vi "Write Command.vi"(8 "Error In":errorcluster, 10 "Command":string, 11 "SerialComm in":refnum<class "SerialComm.lvclass">) -> (0 "Error Out":errorcluster, 3 "SerialComm out":refnum<class "SerialComm.lvclass">)   [LabVIEW 2016, in "SerialComm.lvclass"]
uses:
  SerialComm.lvclass
  SerialComm.lvclass/SerialComm.ctl
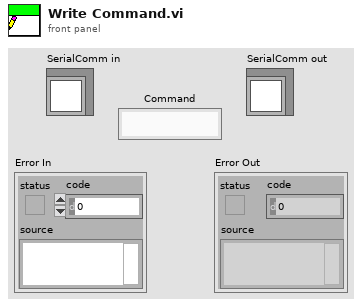
[diagram p1: front panel]
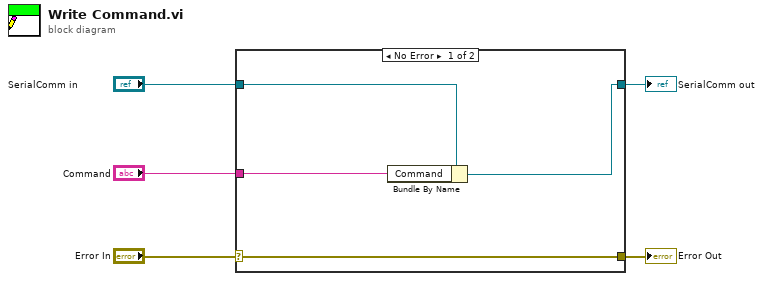
[diagram p0: block diagram]
diagram:
  n1 = case shown="No Error" "Error In" {
    selector: "Error In" -> [w9 w10]
    tunnel: [w9 w10] -> w4
    tunnel: [w7 w11] -> w2
    tunnel: "SerialComm in" -> [w8 w11]
    tunnel: "Command" -> [w6 _]
    frame No Error {
      n2 = Bundle By Name(cluster=w8, "Command"=w6) -> (w7:refnum<class "SerialComm.lvclass">)
    }
    frame Error {
    }
  }
  "Error Out" <- w4
  "SerialComm out" <- w2
